vi "settemp.vi"(2 "Read":bool, 3 "Write":bool=TRUE, 4 "error in":errorcluster, 6 "Characters to Write":string, 7 "GPIB\nAddress":string="1") -> (0 "error out":errorcluster)   [LabVIEW 2025]
doc: "A device connected to a GPIB bus can be written to or be read from using this VI. Select the GPIB address of the device, choose Read or Write or both, type in the characters to be written, and run the VI. If you choose both Read and Write, the VI will write to the device first, then read from the device. Before using this VI you should initialize the GPIB address according to the device's specifications with the \"GPIB Initialization\" function.\nAuthor: Scott Hannahs <sth@magnet.fsu.edu>\n\nThis software is licensed for use under the “MIT License\"\nCopyright (c) 2025 Scott Hannahs, sth@sth@magnet.sthnet.net\n\nPermission is hereby granted, free of charge, to any person obtaining a copy of this software and associated documentation files (the \"Software\"), to deal in the Software without restriction, including without limitation the rights to use, copy, modify, merge, publish, distribute, sublicense, and/or sell copies of the Software, and to permit persons to whom the Software is furnished to do so, subject to the following conditions: The above copyright notice and this permission notice shall be included in all copies or substantial portions of the Software.\n\nTHE SOFTWARE IS PROVIDED \"AS IS\", WITHOUT WARRANTY OF ANY KIND, EXPRESS OR IMPLIED, INCLUDING BUT NOT LIMITED TO THE WARRANTIES OF MERCHANTABILITY, FITNESS FOR A PARTICULAR PURPOSE AND NONINFRINGEMENT. IN NO EVENT SHALL THE AUTHORS OR COPYRIGHT HOLDERS BE LIABLE FOR ANY CLAIM, DAMAGES OR OTHER LIABILITY, WHETHER IN AN ACTION OF CONTRACT, TORT OR OTHERWISE, ARISING FROM, OUT OF OR IN CONNECTION WITH THE SOFTWARE OR THE USE OR OTHER DEALINGS IN THE SOFTWARE."
panel:
  out "Characters Read":string
  out "Write Status":string
  out "Read Status":string
  in  "# bytes\nto read":i32=200
  # "Select  the GPIB address of the device, choose Read or Write or both, type in the characters to be written, and run the VI. If you choose both Read and Write, the VI will write to the device first, then read from the device.  Before using this VI, you should consider initializing the bus with the \"GPIB Initialization\" function."
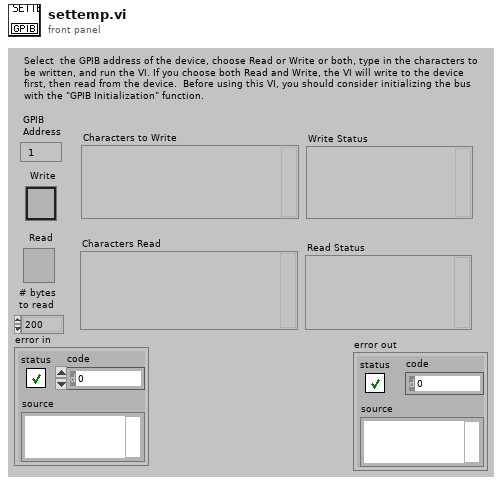
[diagram p1: front panel]
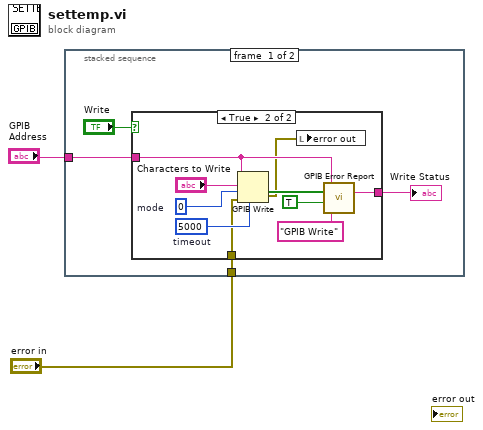
[diagram p0: block diagram]
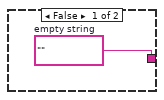
[diagram p2: hidden frame]
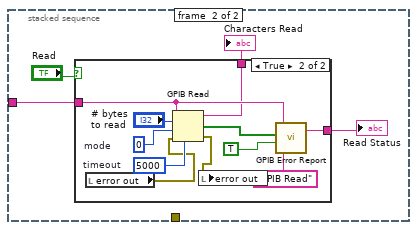
[diagram p3: hidden frame]
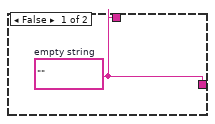
[diagram p4: hidden frame]
diagram:
  n1 = stacked-sequence {
    tunnel: "GPIB\nAddress" -> [w6 w21]
    tunnel: "error in" -> [w3 _]
    frame #0 {
      n2 = case shown="True" "Write" {
        tunnel: [w7 w11] -> w4
        tunnel: w6 -> [_ w15]
        tunnel: w3 -> [_ w9]
        frame False {
          w7 = ""  # empty string
        }
        frame True {
          w17 = 0  # mode
          w10 = u32 5000  # timeout
          n3 = GPIB Write(0:w15, 1:"Characters to Write", 2:w17, 3:w9, 4:w10) -> (5:w14:bool[], 6:w8:errorcluster)
          n4 = local write "error out"(w8) -> ()
          n5 = call "GPIB Error Report.vi"("Function"="GPIB Write", "Dialog?(F)"=TRUE, "Status"=w14, "Address String"=w15) -> ("Status String"=w11:string)  [unwired: 1 out]
        }
      }
      "Write Status" <- w4
    }
    frame #1 {
      n6 = case shown="True" "Read" {
        tunnel: [w22 w27] -> w18
        tunnel: [w22 w28] -> w19
        tunnel: w21 -> [_ w32]
        frame False {
          w22 = ""  # empty string
        }
        frame True {
          w26 = u32 5000  # timeout
          w33 = 0  # mode
          n7 = local read "error out"() -> (w24:errorcluster)
          n8 = GPIB Read(0:w32, 1:"# bytes\nto read", 2:w33, 3:w24, 4:w26) -> (5:w27:string, 6:w25:bool[], 7:w23:errorcluster)
          n9 = local write "error out"(w23) -> ()
          n10 = call "GPIB Error Report.vi"("Function"="GPIB Read", "Dialog?(F)"=TRUE, "Status"=w25, "Address String"=w32) -> ("Status String"=w28:string)  [unwired: 1 out]
        }
      }
      "Characters Read" <- w18
      "Read Status" <- w19
    }
  }
